vi "Initialize Async VIs.vi"(6 "VI in":refnum<vi>, 8 "error in (no error)":errorcluster, 10 "Async VI Parameters":variant[](array[variant]), 11 "Async VI Refs":refnum<vi>[](array[refnum])) -> (0 "error out":errorcluster, 2 "Error Handling Refs":T1, 3 "Async VI Refs out":refnum<vi>[](array[refnum]))   [LabVIEW 2013, in "Diagnostics Addon Engine.lvlib" / "Inline Async API.lvlib"]
uses:
  Inline Async API.lvlib
  Error Handling API/Controls/Error Handling Cluster.ctl
  Controls/Parameters Cluster.ctl
  Error Handling API/Error Handling API.lvlib
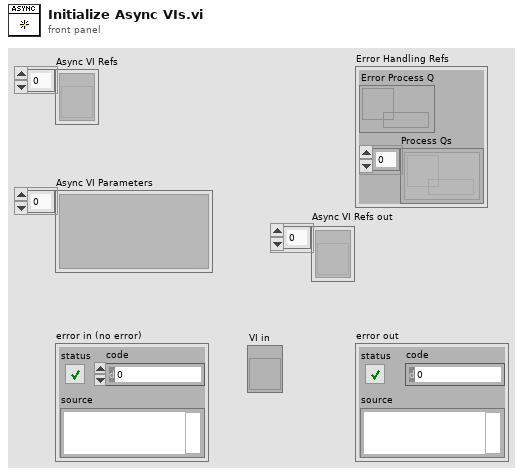
[diagram p1: front panel]
types:
  T1 = typedef "Diagnostics Addon Engine.lvlib/Error Handling API.lvlib/Error Handling Cluster.ctl" = cluster{"Error Process Q":refnum<queue>, "Process Qs":refnum<queue>[]}
  T2 = typedef "Diagnostics Addon Engine.lvlib/Inline Async API.lvlib/Parameters Cluster.ctl" = cluster{"Parameter Name":string, "Initial Settings":variant}
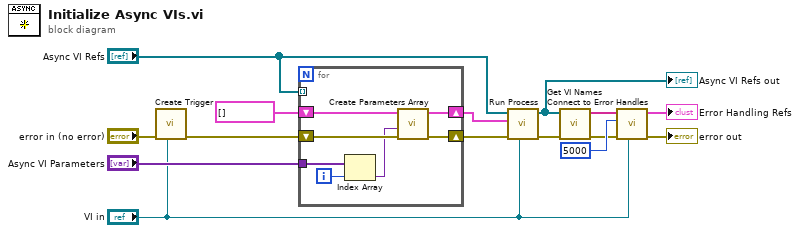
[diagram p0: block diagram]
diagram:
  n1 = call "Create Trigger.vi"("This VI"="VI in", "error in (no error)"="error in (no error)") -> ("error out"=w9:errorcluster)  [unwired: 9 in]
  n2 = for {
    shift-right: [w22] -> w8
    shift-left: cluster{T2[]}[] [] ("Initial Parameters") -> [w19]
    shift-right: [w20] -> w10
    shift-left: w9 -> [w21]
    tunnel: "Async VI Refs" -> [_] mode=indexing
    tunnel: "Async VI Parameters" -> [w17]
    i -> [w18]
    n3 = Index Array(array=w17, index=w18) -> (element=w16:variant)
    n4 = call "Create Parameters Array.vi"("error in (no error)"=w21, "Initial Settings"=w16, "Initial Parameters"=w19) -> ("error out"=w20:errorcluster, "Initial Parameters"=w22:cluster{T2[]}[])  [unwired: 7 in]
  }
  n5 = call "Run Process.vi"("Parent VI"="VI in", "error in (no error)"=w10, "Initial Parameters"=w8, "VI Ref In"="Async VI Refs") -> ("error out"=w3:errorcluster, "VI Ref In"=w2:refnum<vi>[])  [unwired: 6 in]
  "Async VI Refs out" <- w2
  n6 = call "Get VI Names.vi"("error in"=w3, "VI References"=w2) -> ("error out"=w4:errorcluster, "Clone Names"=w5:string[])  [unwired: 8 in]
  n7 = call "Connect to Error Handles.vi"("Parent"="VI in", "error in"=w4, "Timeout (ms)"=u16 5000, "Process Names"=w5) -> ("error out"=→"error out":errorcluster, "Error Handling Cluster"=→"Error Handling Refs":T1)  [unwired: 6 in]
